vi "Add Active DUT Connector Band.vi"(5 "Bands":cluster{"Type (LTE)":i32, "Band Number":i32}[](array[cluster]) {"Type (LTE)" items=["LTE", "New Radio", "WLAN"]}, 7 "RX (RX0)":i32(ring) items=["RX0", "RX1", "RX2", "RX3", "None"], 8 "error in (no error)":errorcluster, 9 "TX (TX0)":i32(ring) items=["TX0", "TX1", "None"], 10 "Connector (\"Connector1\")":string="Connector1", 11 "VISA resource name":refnum<visa-resource-name>) -> (0 "error out":errorcluster, 3 "VISA resource name out":refnum<visa-resource-name>)   [LabVIEW 2015, in "Rohde&Schwarz CMXP Base.lvlib"]
doc: "Assigns frequency bands to a single antenna connector of the active DUT (connector-centric approach).\n\nYou can assign several bands with a single command. Specify the technology and the band number for each band.\n\nAttribute:\n-\n\nRemote-control command:\nADD:DUT:CONNector:BAND"
uses:
  <instrlib>/Rohde&Schwarz CMXP Base/Rohde&Schwarz CMXP Base.lvlib
  <instrlib>/Rohde&Schwarz CMXP Base/Private/rsidr_core.llb/rsidr_core.lvlib
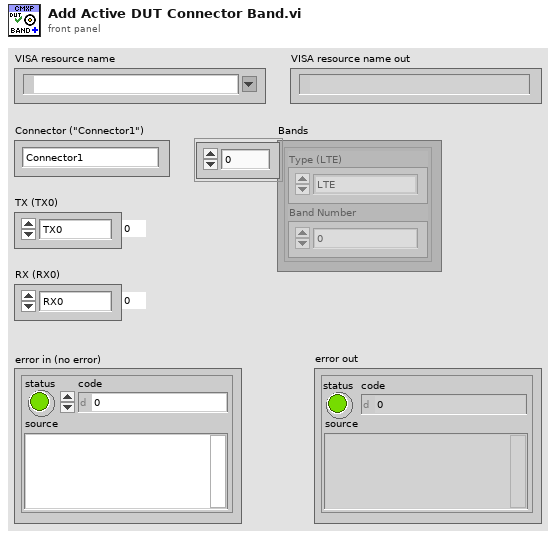
[diagram p1: front panel]
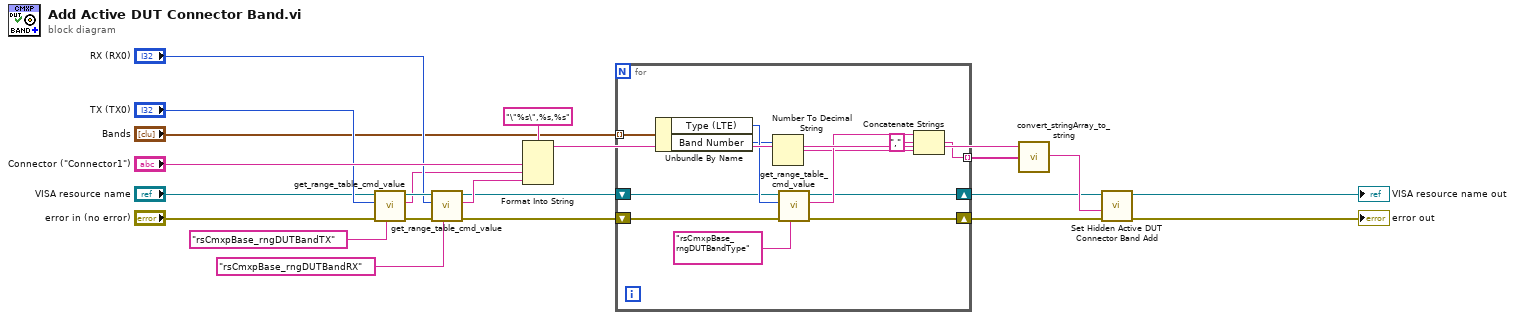
[diagram p0: block diagram]
diagram:
  n1 = call <instrlib>:"get_range_table_cmd_value.vi"("Range Table ID in"="rsCmxpBase_rngDUTBandTX", "error in"="error in (no error)", "Input Int32 value"="TX (TX0)", "VISA resource name"="VISA resource name") -> ("error out"=w20:errorcluster, "Cmd value out"=w9:string, "VISA resource name out"=w19:refnum<visa-resource-name>)  [unwired: 5 in]
  n2 = call <instrlib>:"get_range_table_cmd_value.vi"("Range Table ID in"="rsCmxpBase_rngDUTBandRX", "error in"=w20, "Input Int32 value"="RX (RX0)", "VISA resource name"=w19) -> ("error out"=w4:errorcluster, "Cmd value out"=w8:string, "VISA resource name out"=w3:refnum<visa-resource-name>)  [unwired: 5 in]
  n3 = Format Into String(format string="\"%s\",%s,%s", "Connector (\"Connector1\")", w9, w8) -> (resulting string=w7:string)  [unwired: 2 in, 1 out]
  n4 = for {
    tunnel: "Bands" -> [w34] mode=indexing
    tunnel: [w31] -> w6 mode=indexing
    shift-right: [w23] -> w1
    shift-left: w3 -> [w25]
    shift-right: [w24] -> w2
    shift-left: w4 -> [w26]
    n5 = Unbundle By Name(w34) -> ("Type (LTE)"=w33:i32, "Band Number"=w28:i32)
    n6 = Number To Decimal String(number=w28) -> (decimal integer string=w27:string)  [unwired: 1 in]
    n7 = call <instrlib>:"get_range_table_cmd_value.vi"("Range Table ID in"="rsCmxpBase_rngDUTBandType", "error in"=w26, "Input Int32 value"=w33, "VISA resource name"=w25) -> ("error out"=w24:errorcluster, "Cmd value out"=w30:string, "VISA resource name out"=w23:refnum<visa-resource-name>)  [unwired: 5 in]
    n8 = Concatenate Strings(w30, "," ("string"), w27) -> (w31:string)
  }
  n9 = call <instrlib>:"convert_stringArray_to_string.vi"("string array in"=w6, "String to add before (\"\")"=w7) -> ("string out"=w5:string)  [unwired: 3 in]
  n10 = call "Set Hidden Active DUT Connector Band Add"("error in (no error)"=w2, "Hidden Active DUT Connector Band Add ()"=w5, "instrument handle"=w1) -> ("error out"=→"error out":errorcluster, "instrument handle out"=→"VISA resource name out":refnum<visa-resource-name>)  [unwired: 7 in]
